vi "Frequency Response Function (Real-Im) 1-1.vi"(0 "time signal X":waveform(dbl), 1 "restart averaging (F)":bool, 2 "window parameter":dbl=nan, 5 "time signal Y":waveform(dbl), 7 "window":T2=1 items=["Rectangle"=0, "Hanning"=1, "Hamming"=2, "Blackman-Harris"=3, "Exact Blackman"=4, "Blackman"=5, "Flat Top"=6, "4 Term B-Harris "=7, "7 Term B-Harris"=8, "Low Sidelobe"=9, "Blackman Nuttall"=11, "Triangle"=30, "Bartlett-Hanning"=31, "Bohman"=32, "Parzen"=33, "Welch"=34, "Kaiser"=60, "Dolph-Chebyshev"=61, "Gaussian"=62], 11 "error in (no error)":errorcluster, 12 "averaging parameters":T3={"averaging mode"=enum."No averaging", "weighting mode"=enum."Exponential", "number of averages"=10} {"number of averages" min=1}, 13 "FRF Mode":enum16{"H1", "H2", "H3"}(ring)) -> (3 "averaging done":bool, 4 "real part":cluster{"f0":dbl, "df":dbl, "real part":dbl[]} {"real part" format="%.2p"; "f0" format="%0.2p"; "df" format="%0.2p"}, 6 "imaginary part":T1 {"imaginary part" format="%.2p"; "f0" format="%0.2p"; "df" format="%0.2p"}, 8 "coherence":cluster{"f0":dbl, "df":dbl, "coherence":dbl[]} {"coherence" format="%.2g"; "df" format="%.2p"; "f0" format="%.2p"}, 10 "averages completed":dbl format="%.2p", 15 "error out":errorcluster)   [LabVIEW 2020, in "NI_MAPro.lvlib"]
doc: "Computes the frequency response and the coherence based on the input signals. Results are returned as <B>real part</B>, <B>imaginary part</B>, and <B>coherence</B>."
uses:
  NI_MAPro.lvlib
  windowTd.ctl
  2-chan State.ctl
  NI_AALPro.lvlib
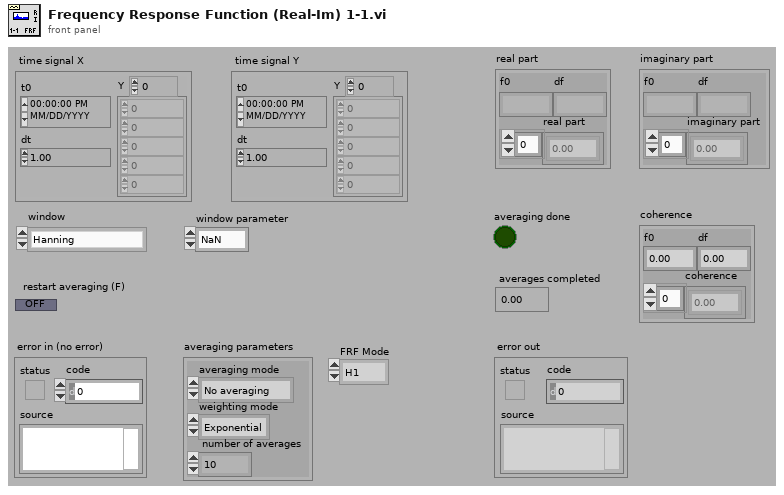
[diagram p1: front panel]
types:
  T1 = cluster{"f0":dbl, "df":dbl, "imaginary part":dbl[]}
  T2 = typedef "NI_AALPro.lvlib/windowTd.ctl" = u32
  T3 = cluster{"averaging mode":enum16{"No averaging", "Vector averaging", "RMS averaging", "Peak hold"}, "weighting mode":enum16{"Linear", "Exponential"}, "number of averages":u32}
  T4 = typedef "NI_MAPro.lvlib/2-chan State.ctl" = cluster{"Sx":cdb[], "Sy":cdb[], "Sxx":dbl[], "Syy":dbl[], "Sxy":cdb[], "block size":i32, "df":dbl, "dt":dbl, "avgs completed":dbl, "spectrum parameters":cluster{"averaging parameters":cluster{"averaging mode":enum16{"No averaging", "Vector averaging", "RMS averaging", "Peak hold"}, "weighting mode":enum16{"Linear", "Exponential"}, "number of averages":u32}, "window":T2}, "lin avg done":bool, "t0 history":dbl, "dt history":dbl, "timestamp":dbl}
  T5 = cluster{"f0":dbl, "df":dbl, "imag or phase":dbl[]}
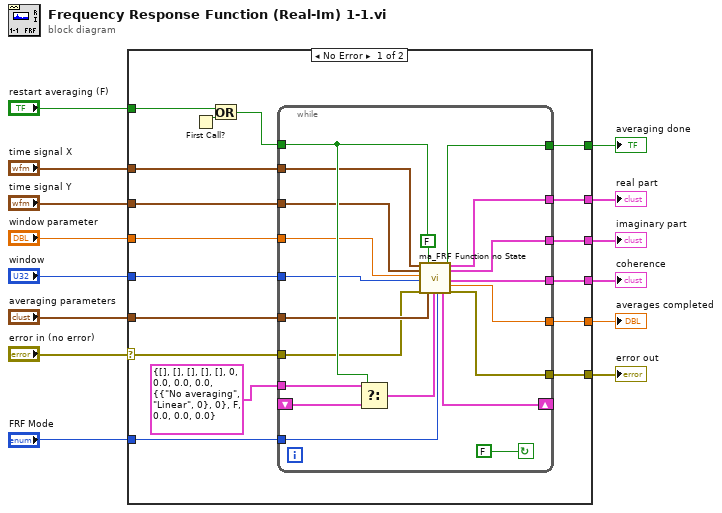
[diagram p0: block diagram]
diagram:
  n1 = case shown="No Error" "error in (no error)" {
    selector: "error in (no error)" -> [w28 w52]
    tunnel: [w29 w52] -> w13
    tunnel: "restart averaging (F)" -> [w26 _]
    tunnel: "time signal X" -> [w25 _]
    tunnel: "time signal Y" -> [w24 _]
    tunnel: "window" -> [w23 _]
    tunnel: "averaging parameters" -> [w22 _]
    tunnel: "FRF Mode" -> [w21 _]
    tunnel: "window parameter" -> [w20 _]
    tunnel: [w19 _] -> w5
    tunnel: [w18 _] -> w4
    tunnel: [w17 _] -> w3
    tunnel: [w16 _] -> w2
    tunnel: [w15 _] -> w1
    frame No Error {
      n2 = First Call?() -> (First Call?: T/F=w31:bool)
      n3 = Or(x=w26, y=w31) -> (x .or. y?=w30:bool)
      n4 = while {
        tunnel: w30 -> [w40]
        tunnel: [w51] -> w19
        tunnel: [w50] -> w15
        tunnel: [w49] -> w18
        tunnel: [w48] -> w29
        shift-right: [w47] -> _
        shift-left: _ -> [w44]
        tunnel: [w42] -> w17
        tunnel: T4 {"Sx"=[], "Sy"=[], "Sxx"=[], "Syy"=[], "Sxy"=[], "block size"=0, "df"=0.0, "dt"=0.0, "avgs completed"=0.0, "spectrum parameters"={"averaging parameters"={"averaging mode"=enum."No averaging", "weighting mode"=enum."Linear", "number of averages"=0}, "window"=0}, "lin avg done"=FALSE, "t0 history"=0.0, "dt history"=0.0, "timestamp"=0.0} ("state info out") -> [w41]
        tunnel: w25 -> [w39]
        tunnel: w24 -> [w38]
        tunnel: w23 -> [w37]
        tunnel: w22 -> [w36]
        tunnel: w21 -> [w35]
        tunnel: [w34] -> w16
        tunnel: w28 -> [w33]
        tunnel: w20 -> [w32]
        stop <- FALSE continue-if-true
        n5 = Select(t=w41, s=w40, f=w44) -> (s? t:f=w45:T4)
        n6 = call "ma_FRF Function no State.vi"("time signal X"=w39, "time signal Y"=w38, "window parameter"=w32, "window"=w37, "error in (no error)"=w33, "restart averaging (F)"=w40, "averaging parameters"=w36, "mag-phase"=FALSE, "state info"=w45, "FRF Mode"=w35) -> ("averaging done"=w51:bool, "state info out"=w47:T4, "real or mag"=w49:cluster{"f0":dbl, "df":dbl, "real or mag":dbl[]}, "imag or phase"=w42:T5, "coherence"=w34:cluster{"f0":dbl, "df":dbl, "coherence":dbl[]}, "averages completed"=w50:dbl, "error out"=w48:errorcluster)  [unwired: 1 in, 2 out]
      }
    }
    frame Error {
    }
  }
  "error out" <- w13
  "averages completed" <- w1
  "averaging done" <- w5
  "coherence" <- w2
  "real part" <- w4
  "imaginary part" <- w3
